vi "Init DI DAQ.vi"(0 "DaqDevice":string="USB6212", 5 "Line":string="port1/line0", 11 "error in":errorcluster) -> (4 "DI task":refnum<k21>, 15 "error out":errorcluster)   [LabVIEW 2017]
doc: "Developed by Kevin Thompson\nThompson Engineering, LLC\nkevin@thompsonengineering.net"
uses:
  <vilib>/DAQmx/create/channels.llb/DAQmx Create Channel (DI-Digital Input).vi
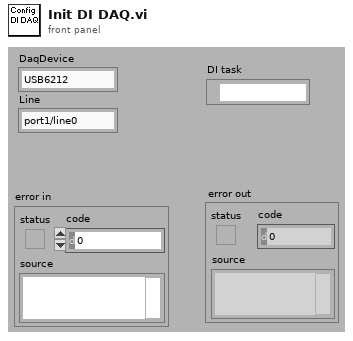
[diagram p1: front panel]
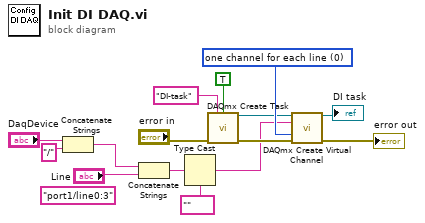
[diagram p0: block diagram]
diagram:
  (unwired) "port1/line0:3"
  w15 = 0 items=["one channel for each line", "one channel for all lines"] ("line grouping")
  n1 = Concatenate Strings("DaqDevice", "/") -> (w7:string)
  n2 = Concatenate Strings(w7, "Line") -> (w13:string)
  n3 = Type Cast(type=tag "" ("lines"), x=w13) -> (*(type *) &x=w8:tag)
  n4 = call <vilib>:"DAQmx Create Task.vi"("new task name"="DI-task", "auto cleanup"=TRUE, "error in"="error in") -> ("task out"=w11:refnum<k21>, "error out"=w10:errorcluster)  [unwired: 11 in]
  n5 = call-poly <vilib>:"DAQmx Create Virtual Channel.vi"("task in"=w11, "lines"=w8, "line grouping"=w15, "error in"=w10) -> ("task out"=→"DI task":refnum<k21>, "error out"=→"error out":errorcluster)  [unwired: 10 in]
